vi "MKS 670 Pressure.vi"(1 "Action":T4=enum."Identify", 2 "Parameters":variant) -> (6 "Output":variant, 7 "Stop":bool)   [LabVIEW 2024]
uses:
  Sub Controls/Instrument Actions.ctl
  Sub Controls/Public.ctl
  Sub Controls/Instrument Match.ctl
  Sub Controls/Factory Reset.ctl
  Sub Controls/Scan Output.ctl
  Sub Controls/Instrument IDN.ctl
  Sub Controls/User Event Command.ctl
panel:
  in  "Factory Reset":T1
  in  "Pressure Sensor Temp(K)":dbl=340.0
  in  "Tube Radius (mm)":dbl=1.2192
  in  "Helium Flavor":u16(ring) items=["Helium-3", "Helium-4"]
  in  "Calc Temperature":bool
  in  "Sensor":enum32{"Chan 1", "Chan 2", "Chan 3"}(radio)
  out "Title":string="MKS 670 Baratron Pressure"
  in  "VISA resource name":refnum<visa-resource-name>
  in  "Instruments":T2[](array[typedef])=[{"Model"="MKS670BD81", "Manufacturer"="MKS Instruments", "Term Character"="", "Wait Time (mS)"=0, "Wait for SRQ"=FALSE, "Type"="Pressure"}]
  out "Model":string
  in  "Address":u16(ring)
  in  "Public":T3
  out "Measurement":dbl[](array[numeric]) format="%^.3e"
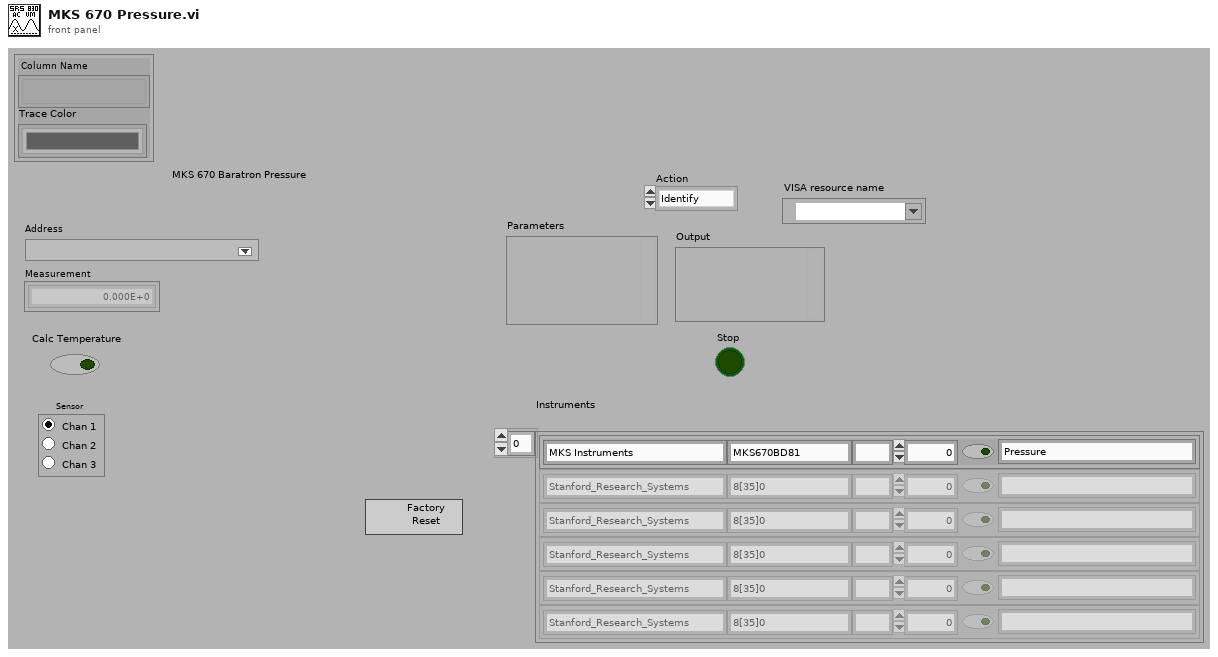
[diagram p1: front panel]
types:
  T1 = typedef "Factory Reset.ctl" = bool
  T2 = typedef "Instrument Match.ctl" = cluster{"Model":string, "Manufacturer":string, "Term Character":string, "Wait Time (mS)":u32, "Wait for SRQ":bool, "Type":string}
  T3 = typedef "Public.ctl" = cluster{"Column Name":string[], "Trace Color":u32[]}
  T4 = typedef "Instrument Actions.ctl" = enum16{"Scan", "Identify", "New", "Configure", "Initialize", "Test", "Read", "Close"}
  T5 = typedef "Scan Output.ctl" = cluster{"Manufacturer":string, "Model":string, "Info":string, "Revision":string, "error out":errorcluster}
  T6 = typedef "Instrument IDN.ctl" = cluster{"VISA Address":string, "Status":u16, "Manufacturer":string, "Model":string, "Info":string, "Info 2":string, "Misc Data":variant}
  T7 = typedef "User Event Command.ctl" = enum32{"Stop Config"}
  T8 = cluster{"VISA resource name":refnum<visa-resource-name>, string}
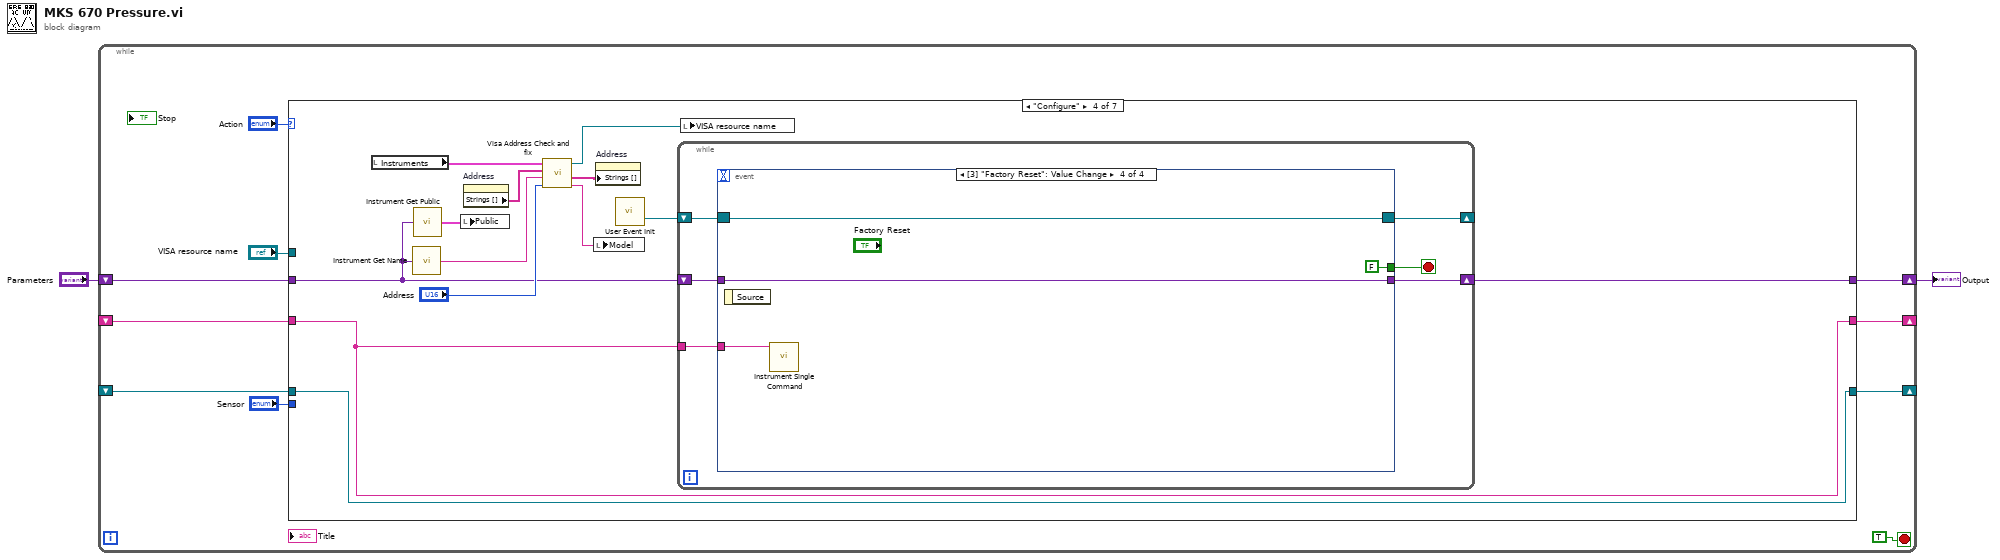
[diagram p0: block diagram]
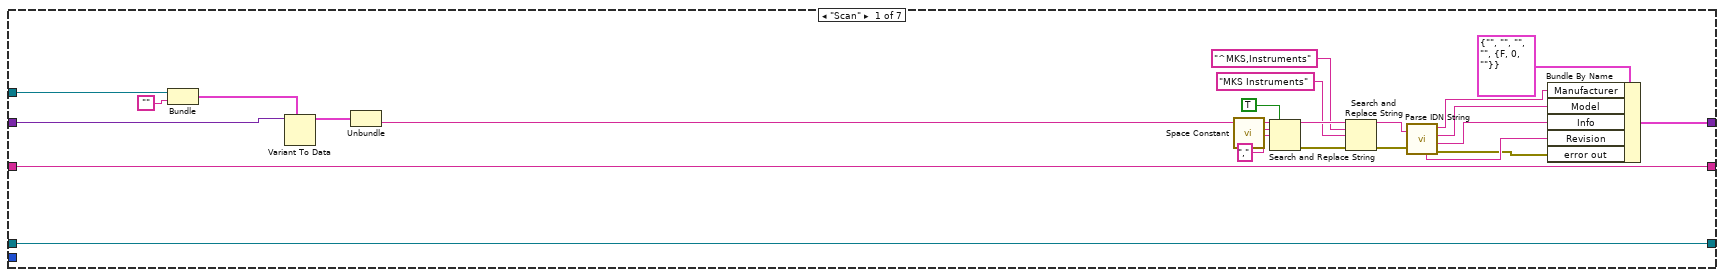
[diagram p2: hidden frame]
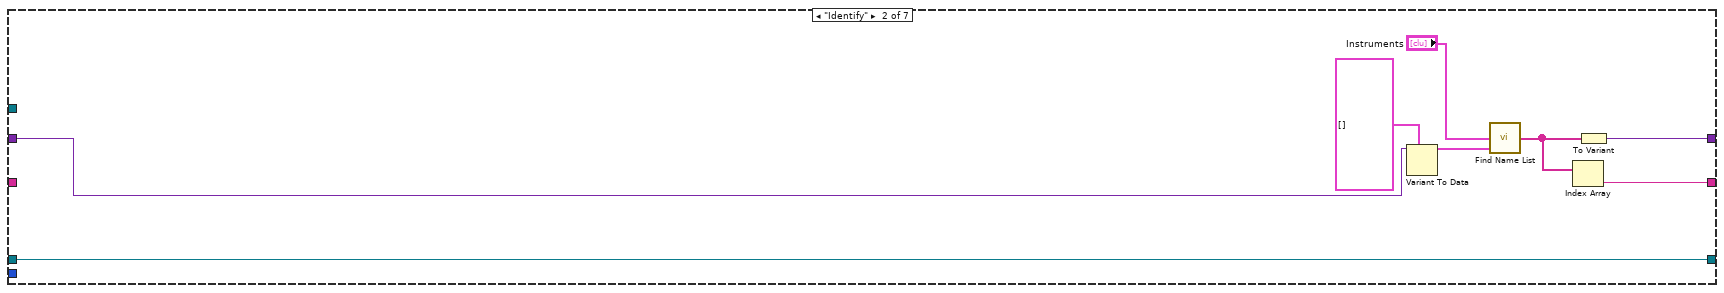
[diagram p3: hidden frame]
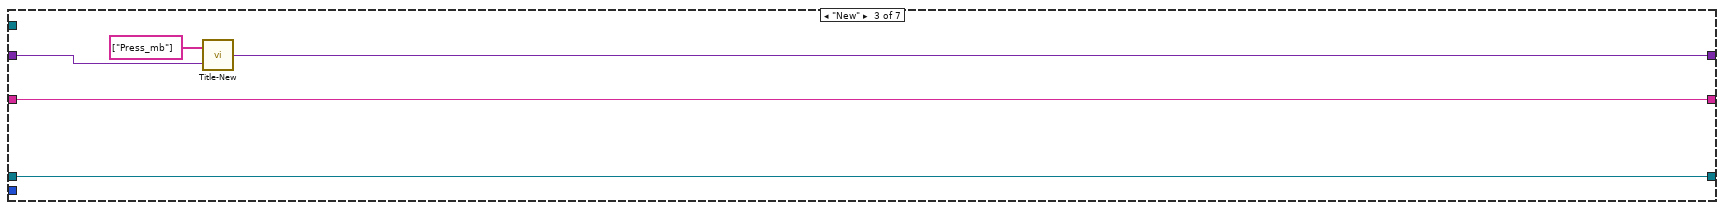
[diagram p4: hidden frame]
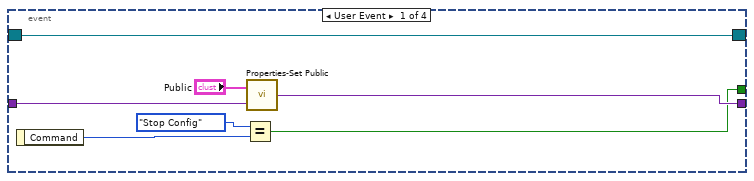
[diagram p5: hidden frame]
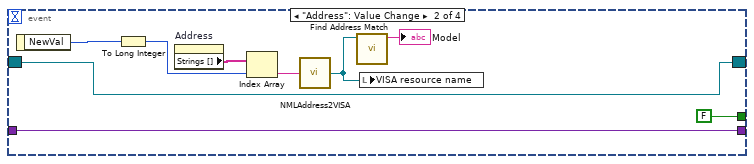
[diagram p6: hidden frame]
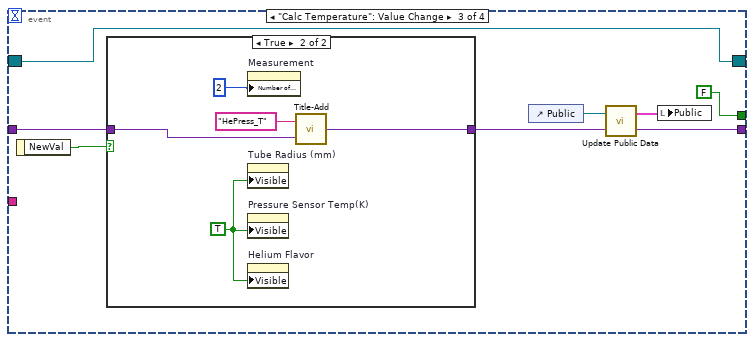
[diagram p7: hidden frame]
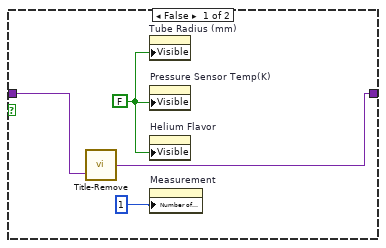
[diagram p8: hidden frame]
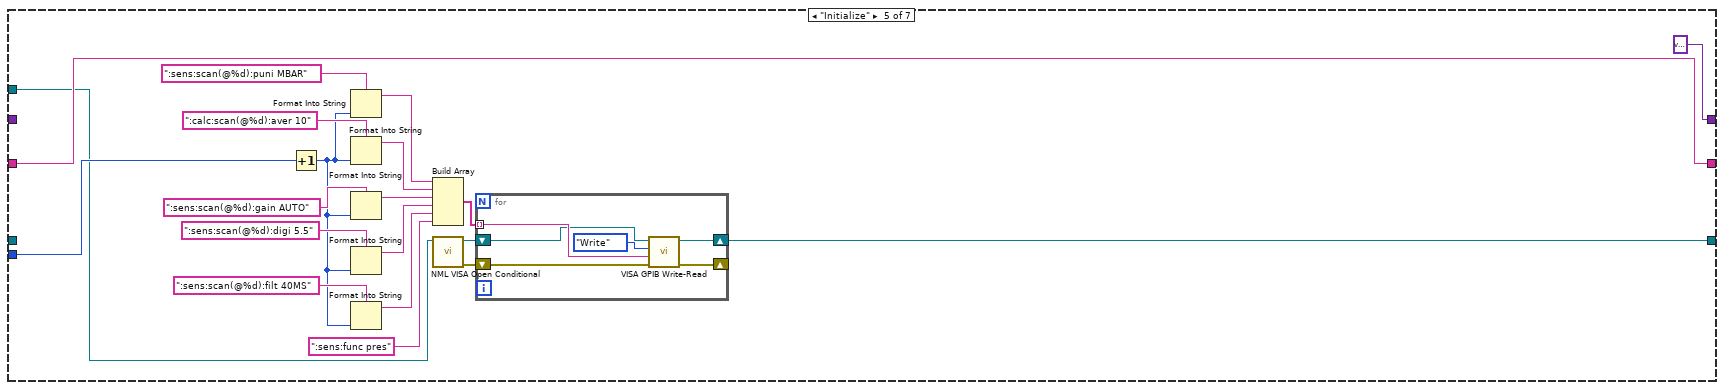
[diagram p9: hidden frame]
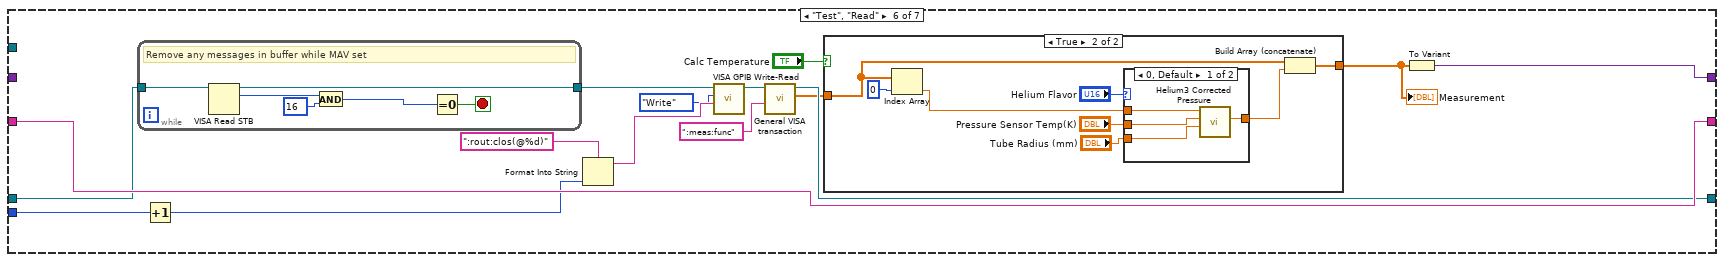
[diagram p10: hidden frame]
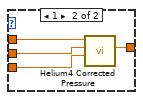
[diagram p12: hidden frame]
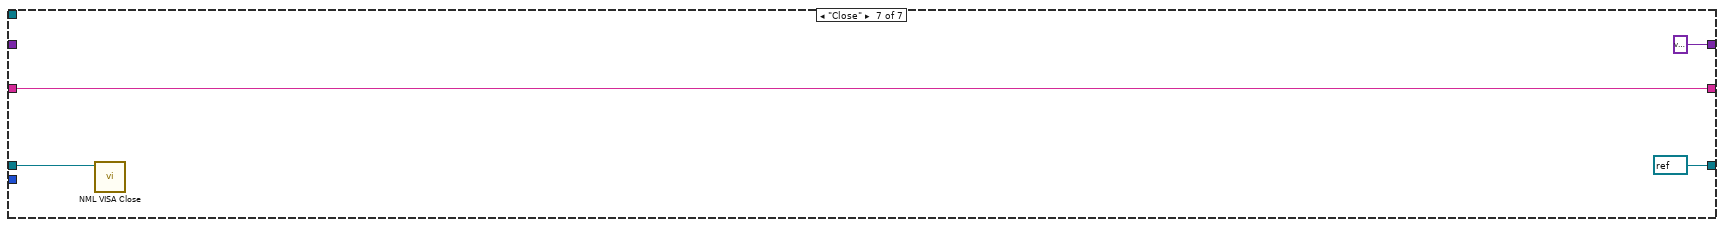
[diagram p13: hidden frame]
diagram:
  n1 = while {
    shift-right: [w11] -> _
    shift-left: _ -> [w10]
    shift-right: [w8] -> w1
    shift-left: "Parameters" -> [w9]
    shift-right: [w5] -> _
    shift-left: _ -> [w4]
    stop <- TRUE stop-if-true
    n2 = case shown="\"Configure\"" "Action" {
      tunnel: [w36 w44 w48 w62 w118 w138 refnum<visa-resource-name> refnum ("Open VISA Resource name")] -> w11
      tunnel: w10 -> [w36 w44 w48 w62 _ w137 w170]
      tunnel: w9 -> [w31 w41 w49 w52 _ _ _]
      tunnel: [w22 w43 w46 w61 variant ("Variant") w146 variant ("Variant")] -> w8
      tunnel: "VISA resource name" -> [w33 _ _ _ w108 _ _]
      tunnel: [w35 w37 w45 w50 w124 w145 w171] -> w5
      tunnel: w4 -> [w35 _ w45 w50 w124 w145 w171]
      tunnel: "Sensor" -> [_ _ _ _ w122 w135 _]
      frame "Scan" {
        n3 = Bundle("VISA resource name"=w33, "") -> (w32:T8)  [unwired: 1 in]
        n4 = Variant To Data(type=w32, Variant=w31) -> (data=w30:T8)  [unwired: 1 in, 1 out]
        n5 = Unbundle(w30) -> (w29:string)  [unwired: 1 out]
        n6 = call <vilib>:"Space Constant.vi"() -> ("String"=w28:string)
        n7 = Search and Replace String(replace all?=TRUE ("replace all? (F)"), input string=w29, search string=w28, replace string="," ("replace string (\"\")")) -> (result string=w27:string, error out=w24:errorcluster)  [unwired: 4 in, 2 out]
        n8 = Search and Replace String(input string=w27, search string="^MKS,Instruments", replace string="MKS Instruments" ("search string"), error in=w24) -> (result string=w16:string, error out=w15:errorcluster)  [unwired: 4 in, 2 out]
        n9 = call "Parse IDN String.vi"("error in (no error)"=w15, "IDN String"=w16) -> ("error out"=w14:errorcluster, "Info"=w18:string, "Model"=w19:string, "Manufacturer"=w20:string, "Revision"=w17:string)
        n10 = Bundle By Name(cluster=T5 {"Manufacturer"="", "Model"="", "Info"="", "Revision"="", "error out"={"status"=FALSE, "code"=0, "source"=""}} ("Scan Output"), "Manufacturer"=w20, "Model"=w19, "Info"=w18, "Revision"=w17, "error out"=w14) -> (w22:T5)
      }
      frame "Identify" {
        n11 = Variant To Data(type=T6[] [], Variant=w41) -> (data=w39:T6[])  [unwired: 1 in, 1 out]
        n12 = call "Find Name List.vi"("Bus Scan"=w39, "Instruments"="Instruments") -> ("Names"=w38:string[])  [unwired: 1 in]
        n13 = Index Array(array=w38) -> (element=w37:string)  [unwired: 1 in]
        n14 = To Variant(anything=w38) -> (Variant=w43:variant)
      }
      frame "New" {
        n15 = call "Title-New.vi"("Parameters"=w49, "Array"=string[] ["Press_mb"]) -> ("Instrument Prop"=w46:variant)
      }
      frame "Configure" {
        n16 = local read "Instruments"() -> (w51:T2[])
        n17 = call "Instrument Get Name.vi"("Parameters"=w52) -> ("Type"=w53:string)
        n18 = call "Instrument Get Public.vi"("Variant"=w52) -> ("Public"=w60:T3)
        n19 = local write "Public"(w60) -> ()
        n20 = property on="Address" class="Ring (strict)"() -> ("Strings []"=w57:string[])  [unwired: 2 in, 2 out]
        n21 = call "Visa Address Check and fix.vi"("Address"="Address", "Name"=w53, "NML Addresses"=w57, "Instruments"=w51) -> ("Model"=w54:string, "NML Addresses"=w55:string[], "VISA resource name"=w56:refnum<visa-resource-name>)  [unwired: 3 out]
        n22 = local write "Model"(w54) -> ()
        n23 = property on="Address" class="Ring (strict)"("Strings []"=w55) -> ()  [unwired: 2 in, 2 out]
        n24 = call "User Event Init.vi"() -> ("Event Registration Refnum"=w59:refnum<event-registration>)  [unwired: 14 in, 1 out]
        n25 = while {
          shift-right: [w68] -> w61
          shift-left: w52 -> [w67]
          shift-right: [w64] -> _
          shift-left: w59 -> [w65]
          tunnel: w50 -> [w63]
          stop <- w66 stop-if-true
          n26 = event shown="[3] \"Factory Reset\": Value Change" {
            selector: w65 -> [w69 w84 w88 w102]
            dyn-events: [w69 w84 w88 w102] -> w64
            timeout: _ -> [_ _ _ _]
            tunnel: [w71 FALSE FALSE FALSE] -> w66
            tunnel: w67 -> [w74 w78 w91 w104]
            tunnel: [w75 w78 w89 w104] -> w68
            tunnel: w63 -> [_ _ _ w105]
            event User Event {
              n27 = event-data() -> ("Command"=w73:T7)  [unwired: 1 in]
              n28 = Equal?(x=User_Event_Command."Stop Config", y=w73) -> (x = y?=w71:bool)
              n29 = call "Properties-Set Public.vi"("Variant"=w74, "New Public"="Public") -> ("Variant 2"=w75:variant)
            }
            event "Address": Value Change {
              n30 = event-data() -> ("NewVal"=w82:u16)  [unwired: 1 in]
              n31 = To Long Integer(number=w82) -> (32bit integer=w76:i32)
              n32 = property on="Address" class="Ring (strict)"() -> ("Strings []"=w81:string[])  [unwired: 2 in, 2 out]
              n33 = Index Array(array=w81, index=w76) -> (element=w80:string)
              n34 = call "NMLAddress2VISA.vi"("NML Address"=w80) -> ("VISA resource name"=w77:refnum<visa-resource-name>)
              n35 = call "Find Address Match.vi"("VISA resource name"=w77) -> ("Model"=→"Model":string)  [unwired: 3 in, 3 out]
              n36 = local write "VISA resource name"(w77) -> ()
            }
            event "Calc Temperature": Value Change {
              n37 = event-data() -> ("NewVal"=w92:bool)  [unwired: 1 in]
              n38 = case shown="True" w92 {
                tunnel: w91 -> [w95 w99]
                tunnel: [w94 w98] -> w90
                frame False {
                  w93 = FALSE ("Visible")
                  n39 = call "Title-Remove.vi"("Parameters"=w95) -> ("Variant"=w94:variant)  [unwired: 1 in]
                  n40 = property on="Tube Radius (mm)" class="DigNum (strict)"("Visible"=w93) -> ()  [unwired: 2 in, 2 out]
                  n41 = property on="Pressure Sensor Temp(K)" class="DigNum (strict)"("Visible"=w93) -> ()  [unwired: 2 in, 2 out]
                  n42 = property on="Helium Flavor" class="Ring (strict)"("Visible"=w93) -> ()  [unwired: 2 in, 2 out]
                  n43 = property on="Measurement" class="Arr (strict)"("Number of Columns"=u32 1) -> ()  [unwired: 2 in, 2 out]
                }
                frame True {
                  w97 = TRUE ("Visible")
                  n44 = property on="Measurement" class="Arr (strict)"("Number of Columns"=u32 2) -> ()  [unwired: 2 in, 2 out]
                  n45 = property on="Tube Radius (mm)" class="DigNum (strict)"("Visible"=w97) -> ()  [unwired: 2 in, 2 out]
                  n46 = property on="Pressure Sensor Temp(K)" class="DigNum (strict)"("Visible"=w97) -> ()  [unwired: 2 in, 2 out]
                  n47 = property on="Helium Flavor" class="Ring (strict)"("Visible"=w97) -> ()  [unwired: 2 in, 2 out]
                  n48 = call "Title-Add.vi"("Parameters"=w99, "String"="HePress_T") -> ("Variant"=w98:variant)
                }
              }
              n49 = control-ref of="Public"() -> (w85:refnum<vi>)
              n50 = call "Update Public Data.vi"("Variant In"=w90, "Public 2"=w85) -> ("Variant Out"=w89:variant, "Public"=w86:T3)
              n51 = local write "Public"(w86) -> ()
            }
            event Value Change {
              n52 = event-data() -> ()  [unwired: 1 in, 1 out]
              n53 = call "Instrument Single Command.vi"("VISA Name"=w105) -> ()  [unwired: 10 in, 1 out]
            }
          }
        }
        n54 = local write "VISA resource name"(w56) -> ()
      }
      frame "Initialize" {
        n55 = Increment(x=w122) -> (x+1=w115:enum32{"Chan 1", "Chan 2", "Chan 3"})
        n56 = Format Into String(format string=":sens:scan(@%d):puni MBAR" ("Command"), w115) -> (resulting string=w109:string)  [unwired: 2 in, 1 out]
        n57 = Format Into String(format string=":calc:scan(@%d):aver 10" ("Command"), w115) -> (resulting string=w110:string)  [unwired: 2 in, 1 out]
        n58 = Format Into String(format string=":sens:scan(@%d):gain AUTO" ("Command"), w115) -> (resulting string=w111:string)  [unwired: 2 in, 1 out]
        n59 = Format Into String(format string=":sens:scan(@%d):digi 5.5" ("Command"), w115) -> (resulting string=w112:string)  [unwired: 2 in, 1 out]
        n60 = Format Into String(format string=":sens:scan(@%d):filt 40MS" ("Command"), w115) -> (resulting string=w113:string)  [unwired: 2 in, 1 out]
        n61 = Build Array(w109, w110, w111, w112, w113, ":sens:func pres" ("Command")) -> (w114:string[])
        n62 = call "NML VISA Open Conditional.vi"("VISA resource name"=w108) -> ("error out"=w106:errorcluster, "dup VISA Session"=w107:refnum<visa-resource-name>)  [unwired: 8 in, 1 out]
        n63 = for {
          tunnel: w114 -> [w130] mode=indexing
          shift-right: [w129] -> w118
          shift-left: w107 -> [w127]
          shift-right: [w126] -> _
          shift-left: w106 -> [w128]
          n64 = call "VISA GPIB Write-Read.vi"("error in (no error)"=w128, "Command"=w130, "Action"=enum16{"Write", "Read", "Write & Read"}."Write", "VISA resource name"=w127) -> ("error out"=w126:errorcluster, "dup VISA Session"=w129:refnum<visa-resource-name>)  [unwired: 4 in, 2 out]
        }
      }
      frame "Test", "Read" {
        n65 = while {
          tunnel: w137 -> [w169]
          tunnel: [w168] -> w136
          stop <- w164 stop-if-true
          # "Remove any messages in buffer while MAV set"
          n66 = VISA Read STB(11:w169) -> (2:w167:u16, 3:w168:refnum<visa-resource-name>)  [unwired: 1 in, 1 out]
          n67 = And(x=w167, y=u16 16) -> (x .and. y?=w165:u16)
          n68 = Equal To 0?(x=w165) -> (x = 0?=w164:bool)
        }
        n69 = Increment(x=w135) -> (x+1=w139:enum32{"Chan 1", "Chan 2", "Chan 3"})
        n70 = Format Into String(format string=":rout:clos(@%d)", w139) -> (resulting string=w141:string)  [unwired: 2 in, 1 out]
        n71 = call "VISA GPIB Write-Read.vi"("Command"=w141, "Action"=enum16{"Write", "Read", "Write & Read"}."Write", "VISA resource name"=w136) -> ("dup VISA Session"=w143:refnum<visa-resource-name>)  [unwired: 5 in, 3 out]
        n72 = call "General VISA transaction.vi"("Command String"=":meas:func" ("t"), "VISA Session"=w143) -> ("Measurement"=w133:dbl[], "dup VISA Session"=w138:refnum<visa-resource-name>)  [unwired: 4 in, 4 out]
        n73 = case shown="True" "Calc Temperature" {
          tunnel: w133 -> [w147 w150]
          tunnel: [w147 w149] -> w132
          frame False {
          }
          frame True {
            n74 = Index Array(array=w150, index=0) -> (element=w154:dbl)
            n75 = case shown="0, Default" "Helium Flavor" {
              tunnel: w154 -> [w159 w163]
              tunnel: "Pressure Sensor Temp(K)" -> [w157 w162]
              tunnel: "Tube Radius (mm)" -> [w158 w161]
              tunnel: [w156 w160] -> w148
              frame 0, Default {
                n76 = call "Helium3 Corrected Pressure.vi"("Tube Radius (mm)"=w158, "Warm Temperature (K)"=w157, "He3 Pressure (mbar)"=w159) -> ("Corrected He3 Temperature (K)"=w156:dbl)  [unwired: 7 in, 1 out]
              }
              frame 1 {
                n77 = call "Helium4 Corrected Pressure.vi"("Tube Radius (mm)"=w161, "Warm Temperature (K)"=w162, "He4 Pressure (mbar)"=w163) -> ("Corrected He4 Temperature (K)"=w160:dbl)  [unwired: 7 in, 1 out]
              }
            }
            n78 = Build Array (concatenate)(w150, w148) -> (w149:dbl[])
          }
        }
        "Measurement" <- w132
        n79 = To Variant(anything=w132) -> (Variant=w146:variant)
      }
      frame "Close" {
        n80 = call "NML VISA Close.vi"("VISA resource name"=w170) -> ()  [unwired: 10 in, 1 out]
      }
    }
  }
  "Output" <- w1
